vi "Rotation Autocorrection.vi"(8 "Gyro":dbl, 9 "Enable\nAutocorrect":bool, 11 "Rotation":dbl) -> (3 "Rotation corrected":dbl)   [LabVIEW 2013]
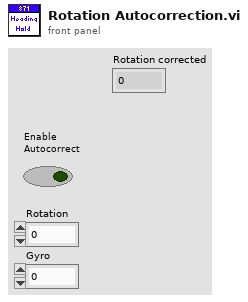
[diagram p1: front panel]
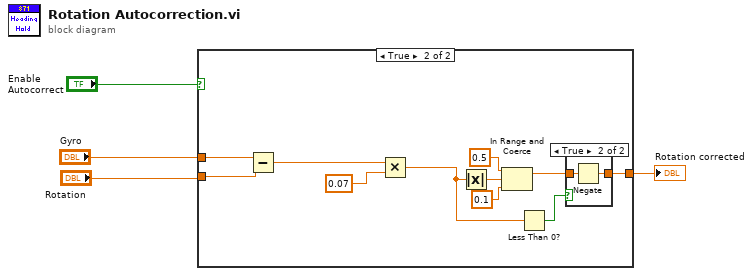
[diagram p0: block diagram]
diagram:
  n1 = case shown="True" "Enable\nAutocorrect" {
    tunnel: "Rotation" -> [w5 w8]
    tunnel: [w5 w11] -> w4
    tunnel: "Gyro" -> [_ w7]
    frame False {
    }
    frame True {
      n2 = Subtract(x=w7, y=w8) -> (x-y=w6:dbl)
      n3 = Multiply(x=w6, y=0.07) -> (x*y=w9:dbl)
      n4 = Absolute Value(x=w9) -> (abs(x)=w14:dbl)
      n5 = In Range and Coerce(upper limit=0.5, x=w14, lower limit=0.1) -> (coerced(x)=w12:dbl)  [unwired: 1 out]
      n6 = Less Than 0?(x=w9) -> (x < 0?=w13:bool)
      n7 = case shown="True" w13 {
        tunnel: w12 -> [w17 w19]
        tunnel: [w17 w18] -> w11
        frame False {
        }
        frame True {
          n8 = Negate(x=w19) -> (-x=w18:dbl)
        }
      }
    }
  }
  "Rotation corrected" <- w4
